vi "Write Wait Until Completion.vi"(8 "error in (no error)":errorcluster, 10 "Wait Until Completion":bool, 11 "CallVIStep in":refnum<class "CallVIStep.lvclass">) -> (0 "error out":errorcluster, 3 "CallVIStep out":refnum<class "CallVIStep.lvclass">)   [LabVIEW 2015, in "CallVIStep.lvclass"]
uses:
  CallVIStep.lvclass
  CallVIStep.lvclass/CallVIStep.ctl
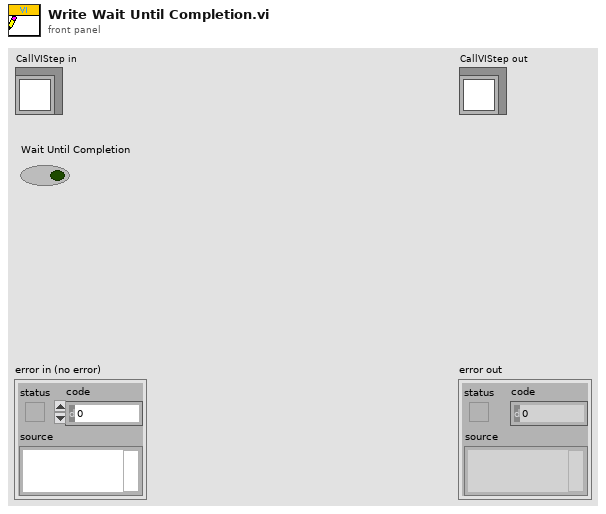
[diagram p1: front panel]
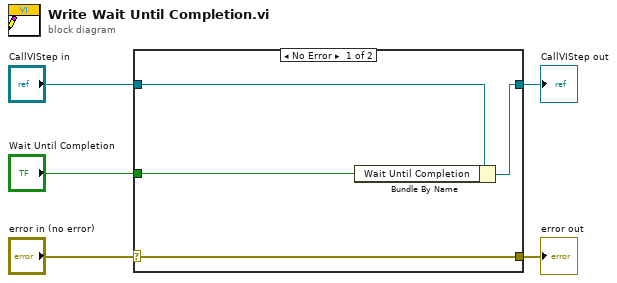
[diagram p0: block diagram]
diagram:
  n1 = case shown="No Error" "error in (no error)" {
    selector: "error in (no error)" -> [w9 w10]
    tunnel: [w9 w10] -> w4
    tunnel: [w7 w11] -> w2
    tunnel: "CallVIStep in" -> [w8 w11]
    tunnel: "Wait Until Completion" -> [w6 _]
    frame No Error {
      n2 = Bundle By Name(cluster=w8, "Wait Until Completion"=w6) -> (w7:refnum<class "CallVIStep.lvclass">)
    }
    frame Error {
    }
  }
  "error out" <- w4
  "CallVIStep out" <- w2
